vi "RF Switch tool by MCU.vi"(5 "Index":i8 min=0 max=24, 6 "array input":bool[][](array[boolean])=array80x96[7680 elements]) -> ()   [LabVIEW 2011]
uses:
  <vilib>/Utility/error.llb/DialogType.ctl
  <vilib>/Utility/file.llb/Read From Spreadsheet File (I64).vi
  <vilib>/Utility/file.llb/Write To Spreadsheet File (I64).vi
panel:
  in  "Index _C":i32[](array[numeric])=[1, 2, 3, 4, 5, 6, 7, 8, 9, 10, 1, 2, 3, 4, 5, 6, 7, 8, 9, 10, 1, 2, 3, 4, 5, 6, 7, 8, 9, 10, 1, 2, 3, 4, 5, 6, 7, 8, 9, 0, 1, 2, 3, 4, 5, 6, 7, 8, 9, 10, 51, 52, 53, 54, 55, 56, 57, 58, 59, 60, 61, 62, 63, 64, 65, 66, 67, 68, 69, 70, 71, 72, 73, 74, 75, 76, 77, 78, 79, 80]
  in  "Index_R":i32[](array[numeric])=[1, 2, 3, 4, 5, 6, 7, 8, 9, 10, 11, 12, 13, 14, 15, 16, 17, 18, 19, 20, 21, 22, 23, 24, 25, 26, 27, 28, 29, 30, 31, 32, 33, 34, 35, 36, 37, 38, 39, 40, 41, 42, 43, 44, 45, 46, 47, 48, 49, 50, 51, 52, 53, 54, 55, 56, 57, 58, 59, 60, 61, 62, 63, 64, 65, 66, 67, 68, 69, 70, 71, 72, 73, 74, 75, 76, 77, 78, 79, 80]
  in  "Function":u16(ring) items=["Testing", "Close All"]
  in  "VISA":refnum<visa-resource-name>="COM3"
  in  "PCI-6509: P0-P1-P2-P3-P4-P5":dbl[](array[numeric])=[1.0, 2.0, 3.0, 4.0, 5.0, 6.0, 7.0, 8.0, 9.0, 10.0, 1.0, 2.0, 3.0, 4.0, 5.0, 6.0, 7.0, 8.0, 9.0, 10.0, 1.0, 2.0, 3.0, 4.0, 5.0, 6.0, 7.0, 8.0, 9.0, 10.0, 1.0, 2.0, 3.0, 4.0, 5.0, 6.0, 7.0, 8.0, 9.0, 10.0, 1.0, 2.0, 3.0, 4.0, 5.0, 6.0, 7.0, 8.0, 9.0, 10.0]
  in  "Switch Matrix":u16(ring)
  in  "Basic Path":path=path "C:/Users/L025200.LUXSHARE/Desktop/VNA Aotomatic Data Save Tool 20150327/Switch Matrix"
  out "Matrix List":string[](array[string])
  out "Path":path=path "C:/Users/L025200.LUXSHARE/Desktop/VNA Aotomatic Data Save Tool 20150327/Switch Matrix"
  in  "Modify":bool
  # "RF Switch Matrix Control System By MCU"
  # "20150714"
  # "-------------Switch1------------"
  # "-------------Switch2------------"
  # "-------------Switch3------------"
  # "-------------Switch4------------"
  # "-------------Switch5------------"
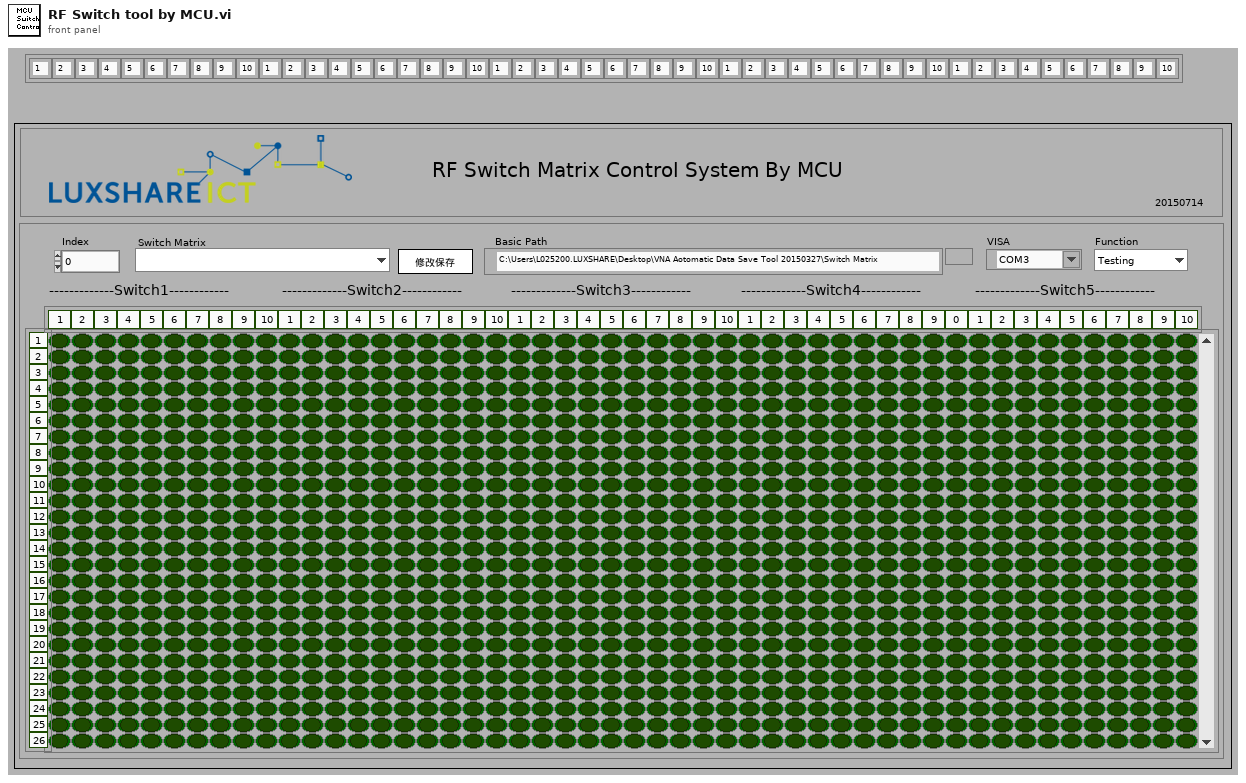
[diagram p1: front panel]
types:
  T1 = typedef "DialogType.ctl" = u16
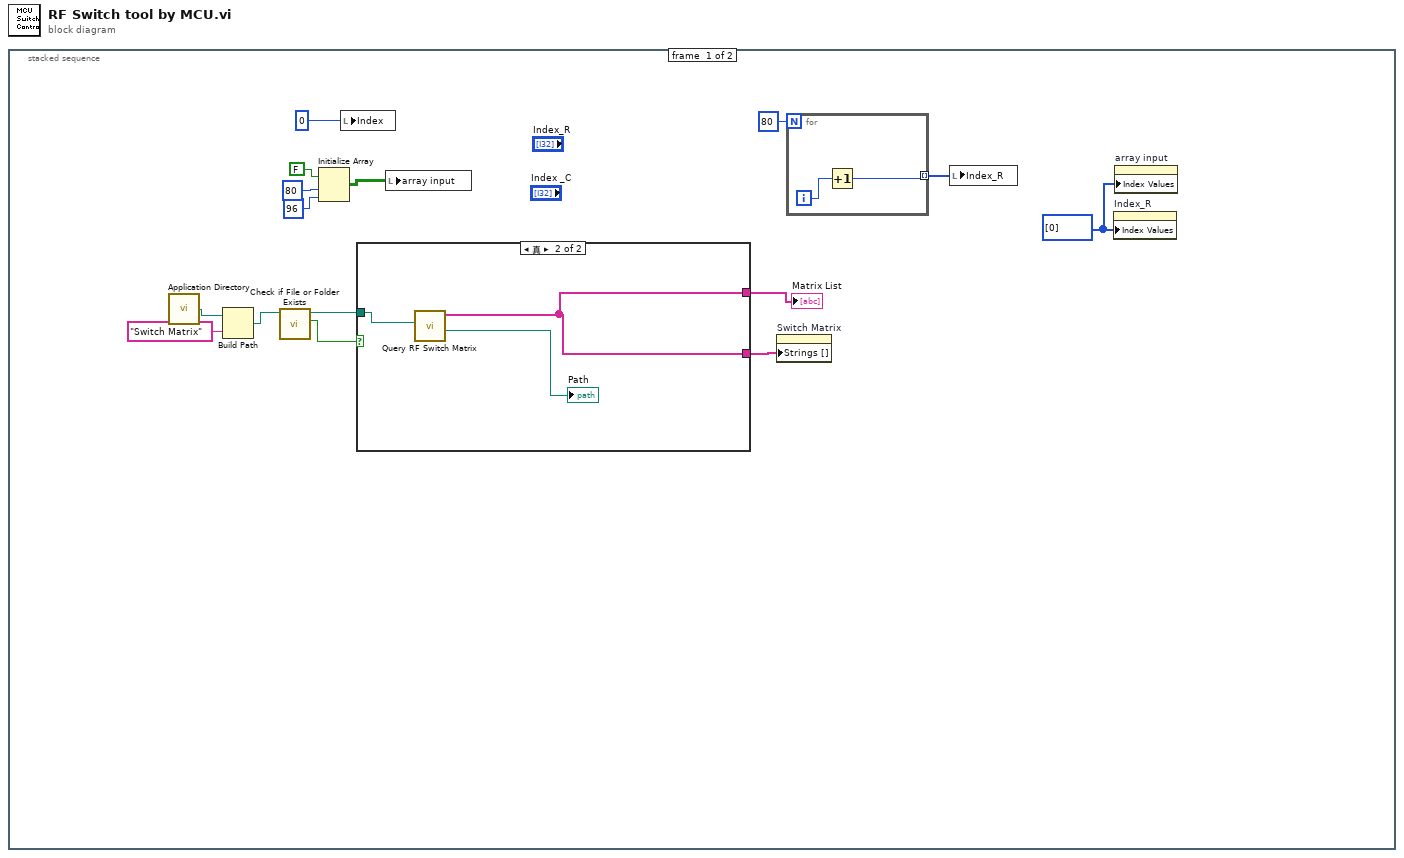
[diagram p0: block diagram]
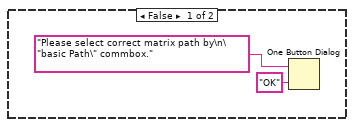
[diagram p2: hidden frame]
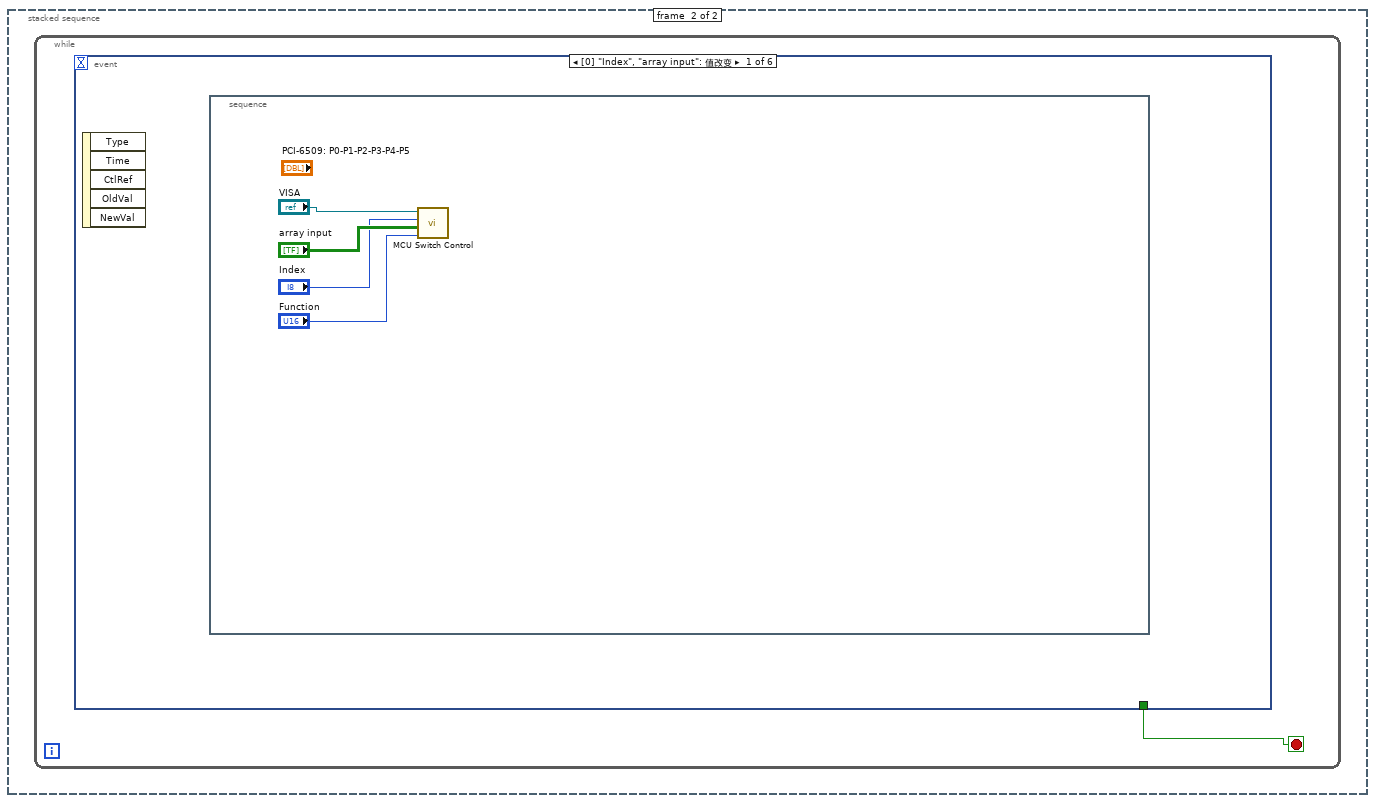
[diagram p3: hidden frame]
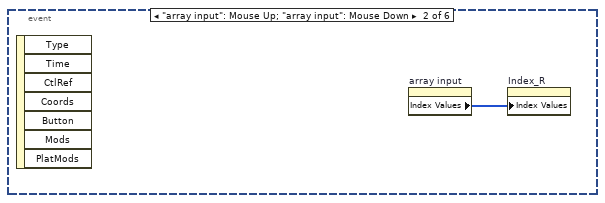
[diagram p4: hidden frame]
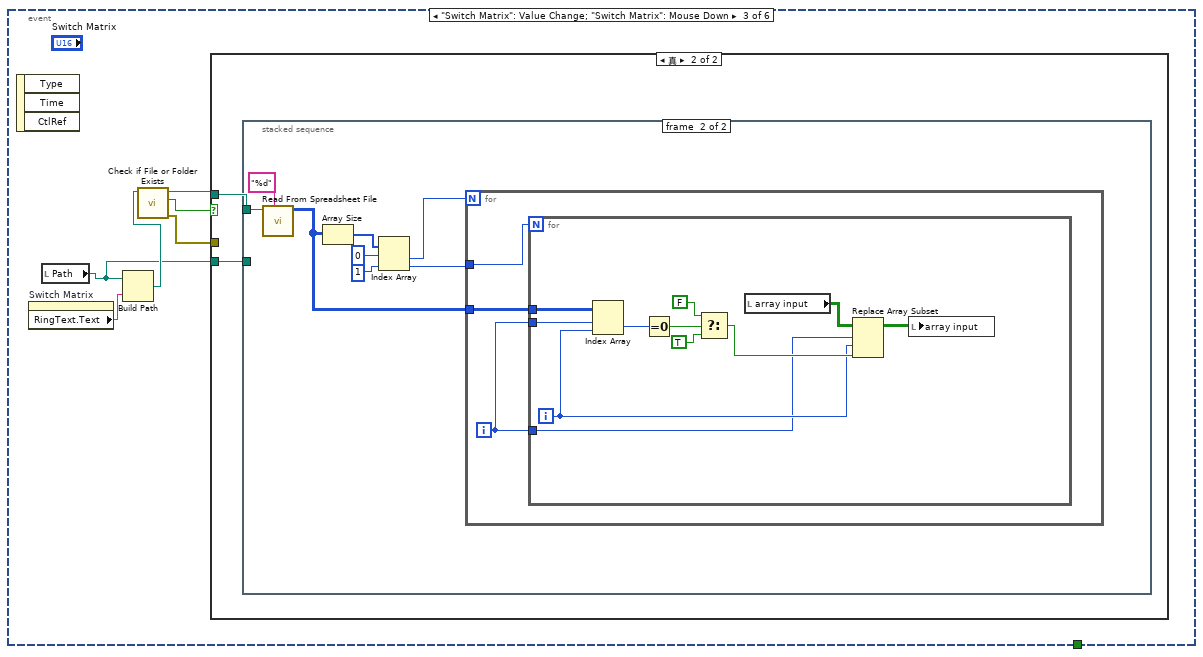
[diagram p5: hidden frame]
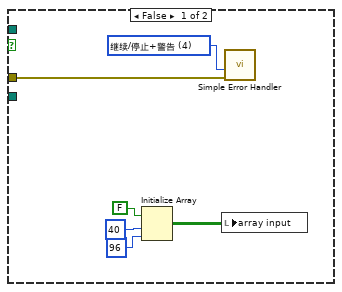
[diagram p6: hidden frame]
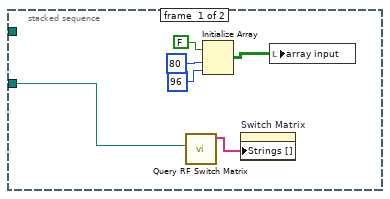
[diagram p7: hidden frame]
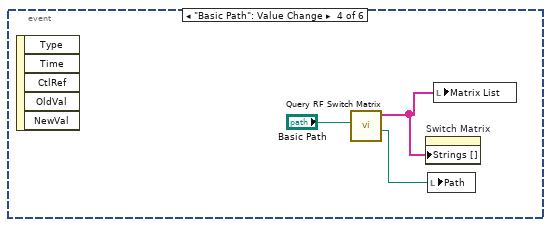
[diagram p8: hidden frame]
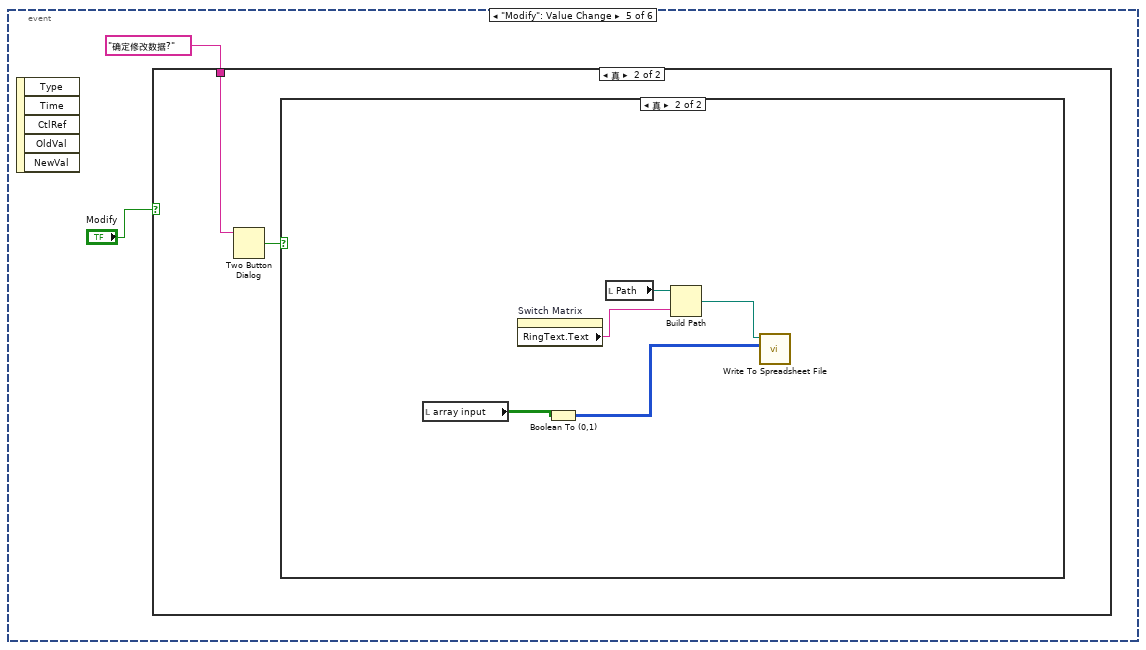
[diagram p9: hidden frame]
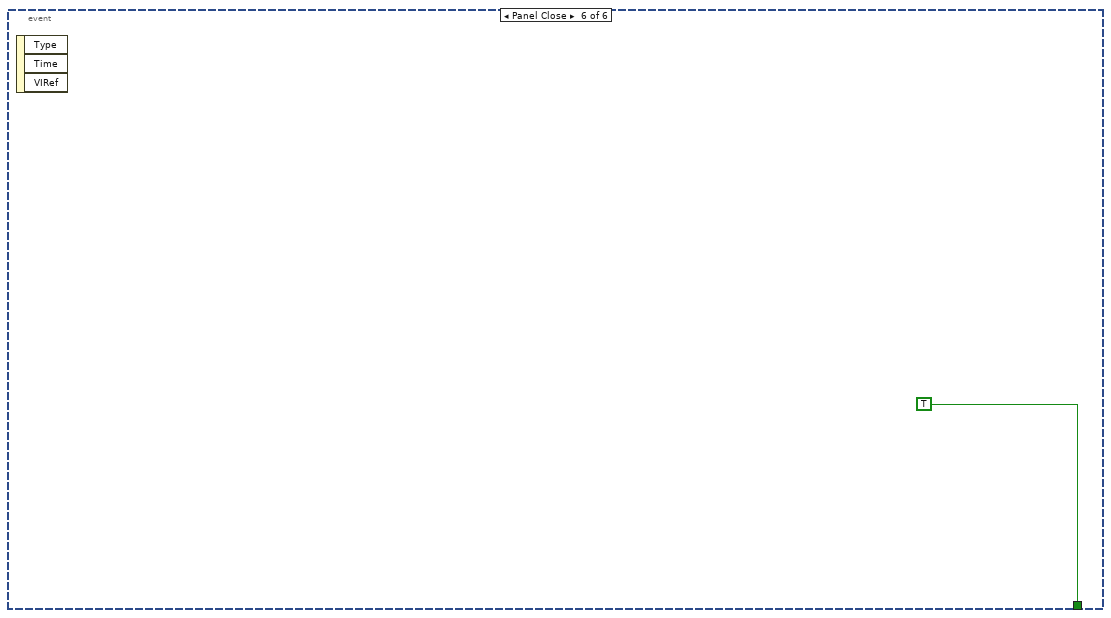
[diagram p12: hidden frame]
diagram:
  n1 = stacked-sequence {
    frame #0 {
      w1 = u32[] [0] ("索引值")
      n2 = call <vilib>:"Application Directory.vi"() -> ("Application Directory"=w10:path)
      n3 = Build Path(base path=w10, name or relative path="Switch Matrix" ("名称或相对路径")) -> (appended path=w8:path)
      n4 = call <vilib>:"Check if File or Folder Exists.vi"("path"=w8) -> ("file or folder exists?"=w7:bool, "dup path"=w6:path)  [unwired: 8 in, 1 out]
      n5 = Initialize Array(FALSE, 80 ("维数大小"), 96 ("维数大小")) -> (w11:bool[][])
      n6 = local write "Index"(i8 0 ("Action Index)")) -> ()
      n7 = case shown="真" w7 {
        tunnel: w6 -> [_ w21]
        tunnel: [_ w20] -> w5
        tunnel: [_ w20] -> w4
        frame False {
          n8 = One Button Dialog(message="Please select correct matrix path by\n\"basic Path\" commbox." ("消息"), button name ("OK")="OK" ("按钮名称（“确定”）")) -> ()  [unwired: 1 out]
        }
        frame True {
          n9 = call "Query RF Switch Matrix.vi"("Basic Path"=w21) -> ("Path"=→"Path":path, "Matrix List"=w20:string[])  [unwired: 9 in]
        }
      }
      "Matrix List" <- w5
      n10 = local write "array input"(w11) -> ()
      n11 = property on="Switch Matrix" class="Ring (严格)"("Strings []"=w4) -> ()  [unwired: 2 in, 2 out]
      n12 = for {
        N: 80 -> [_]
        tunnel: [w16] -> w2 mode=indexing
        i -> [w17]
        n13 = Increment(x=w17) -> (x+1=w16:i32)
      }
      n14 = local write "Index_R"(w2) -> ()
      n15 = property on="Index_R" class="Arr (严格)"("Index Values"=w1) -> ()  [unwired: 2 in, 2 out]
      n16 = property on="array input" class="Arr (严格)"("Index Values"=w1) -> ()  [unwired: 2 in, 2 out]
    }
    frame #1 {
      n17 = while {
        stop <- w23 stop-if-true
        n18 = event shown="[0] \"Index\", \"array input\": 值改变" {
          selector: _ -> [_ _ _ _ _ _]
          dyn-events: _ -> [_ _ _ _ _ _]
          timeout: _ -> [_ _ _ _ _ _]
          tunnel: [_ _ _ _ _ TRUE] -> w23
          event "Index", "array input": Value Change {
            n19 = event-data() -> ()  [unwired: 1 in, 5 out]
            n20 = stacked-sequence {
              frame #0 {
                n21 = call "MCU Switch Control.vi"("Function"="Function", "Array input:"="array input", "Index"="Index", "VISA"="VISA") -> ()  [unwired: 7 in, 1 out]
              }
            }
          }
          event "array input": Mouse Up; "array input": Mouse Down {
            n22 = event-data() -> ()  [unwired: 1 in, 7 out]
            n23 = property on="array input" class="Arr (严格)"() -> ("Index Values"=w28:u32[])  [unwired: 2 in, 2 out]
            n24 = property on="Index_R" class="Arr (严格)"("Index Values"=w28) -> ()  [unwired: 2 in, 2 out]
          }
          event "Switch Matrix": Value Change; "Switch Matrix": Mouse Down {
            n25 = event-data() -> ()  [unwired: 1 in, 3 out]
            n26 = property on="Switch Matrix" class="Ring (严格)"() -> ("RingText.Text"=w34:string)  [unwired: 2 in, 2 out]
            n27 = local read "Path"() -> (w29:path)
            n28 = Build Path(base path=w29, name or relative path=w34) -> (appended path=w33:path)
            n29 = call <vilib>:"Check if File or Folder Exists.vi"("path"=w33) -> ("error out"=w32:errorcluster, "file or folder exists?"=w31:bool, "dup path"=w30:path)  [unwired: 8 in]
            n30 = case shown="真" w31 {
              tunnel: w32 -> [w40 _]
              tunnel: w30 -> [_ w42]
              tunnel: w29 -> [_ w41]
              frame False {
                w39 = T1 4 items=["无对话框", "确定信息", "继续或停止信息", "确定信息＋警告", "继续/停止+警告"] ("type of dialog (OK msg:1)")
                n31 = Initialize Array(FALSE, 40 ("维数大小"), 96 ("维数大小")) -> (w35:bool[][])
                n32 = local write "array input"(w35) -> ()
                n33 = call <vilib>:"Simple Error Handler.vi"("type of dialog (OK msg:1)"=w39, "error in (no error)"=w40) -> ()  [unwired: 3 in, 5 out]
              }
              frame True {
                n34 = stacked-sequence {
                  tunnel: w42 -> [_ w49]
                  tunnel: w41 -> [w44 _]
                  frame #0 {
                    n35 = call "Query RF Switch Matrix.vi"("Basic Path"=w44) -> ("Matrix List"=w43:string[])  [unwired: 9 in, 1 out]
                    n36 = Initialize Array(FALSE, 80 ("维数大小"), 96 ("维数大小")) -> (w45:bool[][])
                    n37 = property on="Switch Matrix" class="Ring (严格)"("Strings []"=w43) -> ()  [unwired: 2 in, 2 out]
                    n38 = local write "array input"(w45) -> ()
                  }
                  frame #1 {
                    n39 = call-poly <vilib>:"Read From Spreadsheet File.vi"("format (%d)"="%d" ("format (%.3f)"), "file path (dialog if empty)"=w49) -> ("all rows"=w56:i64[][])  [unwired: 5 in, 4 out]
                    n40 = Array Size(array=w56) -> (size(s)=w50:i32[])
                    n41 = Index Array(array=w50, index #1=0 ("索引"), index #2=1 ("索引")) -> (element #1=w53:i32, element #2=w54:i32)
                    n42 = for {
                      N: w53 -> [_]
                      tunnel: w54 -> [w59]
                      tunnel: w56 -> [w58]
                      i -> [w57]
                      n43 = for {
                        N: w59 -> [_]
                        tunnel: w58 -> [w70]
                        tunnel: w57 -> [w69]
                        tunnel: w57 -> [w62]
                        i -> [w63]
                        n44 = Index Array(array=w70, index (row)=w69, index (col)=w63) -> (element=w68:i64)
                        n45 = Equal To 0?(x=w68) -> (x = 0?=w67:bool)
                        n46 = Select(t=FALSE, s=w67, f=TRUE) -> (s? t:f=w64:bool)
                        n47 = local read "array input"() -> (w60:bool[][])
                        n48 = Replace Array Subset(array=w60, new element=w64, index (row)=w62, index (col)=w63) -> (w61:bool[][])
                        n49 = local write "array input"(w61) -> ()
                      }
                    }
                  }
                }
              }
            }
          }
          event "Basic Path": Value Change {
            n50 = event-data() -> ()  [unwired: 1 in, 5 out]
            n51 = call "Query RF Switch Matrix.vi"("Basic Path"="Basic Path") -> ("Path"=w72:path, "Matrix List"=w73:string[])  [unwired: 9 in]
            n52 = property on="Switch Matrix" class="Ring (严格)"("Strings []"=w73) -> ()  [unwired: 2 in, 2 out]
            n53 = local write "Path"(w72) -> ()
            n54 = local write "Matrix List"(w73) -> ()
          }
          event "Modify": Value Change {
            n55 = event-data() -> ()  [unwired: 1 in, 5 out]
            n56 = case shown="真" "Modify" {
              tunnel: "确定修改数据?" ("消息") -> [_ w77]
              frame False {
              }
              frame True {
                n57 = Two Button Dialog(message=w77) -> (T button?=w76:bool)  [unwired: 2 in]
                n58 = case shown="真" w76 {
                  frame False {
                  }
                  frame True {
                    n59 = local read "array input"() -> (w82:bool[][])
                    n60 = property on="Switch Matrix" class="Ring (严格)"() -> ("RingText.Text"=w78:string)  [unwired: 2 in, 2 out]
                    n61 = Boolean To (0,1)(Boolean=w82) -> (0, 1=w81:i16[][])
                    n62 = local read "Path"() -> (w79:path)
                    n63 = Build Path(base path=w79, name or relative path=w78) -> (appended path=w80:path)
                    n64 = call-poly <vilib>:"Write To Spreadsheet File.vi"("2D data"=w81, "file path (dialog if empty)"=w80) -> ()  [unwired: 6 in, 1 out]
                  }
                }
              }
            }
          }
          event Panel Close {
            n65 = event-data() -> ()  [unwired: 1 in, 3 out]
          }
        }
      }
    }
  }
